vi "test_CRIO daqmx PWM.vi"() -> ()   [LabVIEW 2023]
uses:
  DIO/DO DAQmx PWM CFG/DO DAQmx PWM CFG.lvclass
  Measure and Stimulus Subsystems/Measure and Stimulus Subsystems.lvclass
  DIO/Virtual DIO/Virt PWM Generator/Virt DAQmx PWM Generator.lvclass
panel:
  out "Iteration":i32
  in  "Stop":bool
  out "Error Out":errorcluster
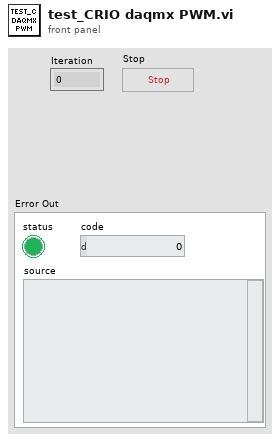
[diagram p1: front panel]
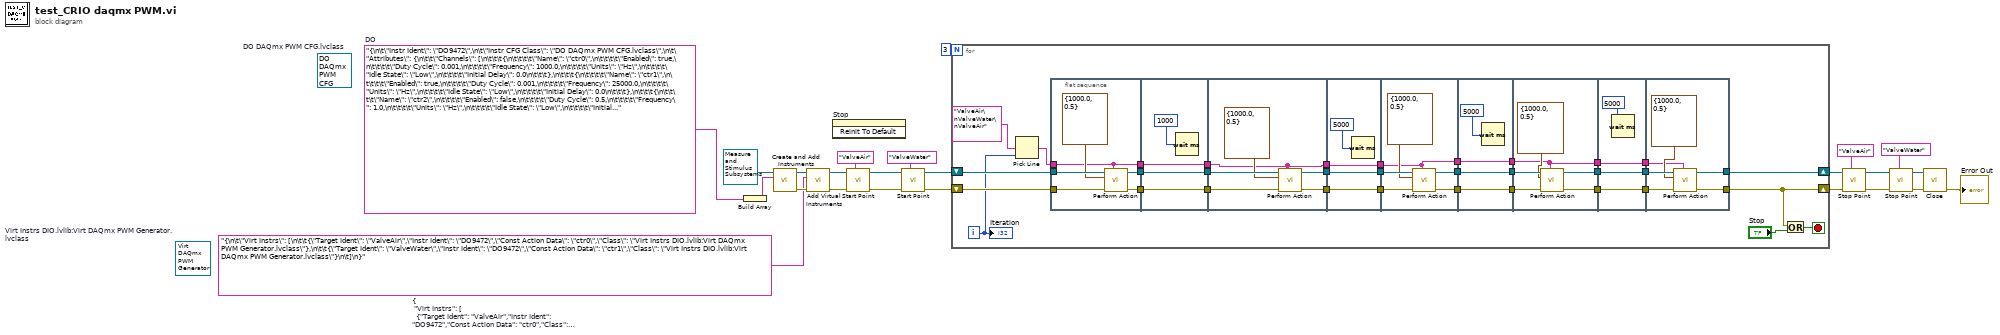
[diagram p0: block diagram]
diagram:
  (unwired) refnum<class "Virt DAQmx PWM Generator.lvclass"> refnum  # Virt Instrs DIO.lvlib:Virt DAQmx PWM Generator.lvclass
  (unwired) refnum<class "DO DAQmx PWM CFG.lvclass"> refnum  # DO DAQmx PWM CFG.lvclass
  w16 = "{\n\t\"Instr Ident\": \"DO9472\",\n\t\"Instr CFG Class\": \"DO DAQmx PWM CFG.lvclass\",\n\t\"Attributes\": {\n\t\t\"Channels\": [\n\t\t\t{\n\t\t\t\t\"Name\": \"ctr0\",\n\t\t\t\t\"Enabled\": true,\n\t\t\t\t\"Duty Cycle\": 0.001,\n\t\t\t\t\"Frequency\": 1000.0,\n\t\t\t\t\"Units\": \"Hz\",\n\t\t\t\t\"Idle State\": \"Low\",\n\t\t\t\t\"Initial Delay\": 0.0\n\t\t\t},\n\t\t\t{\n\t\t\t\t\"Name\": \"ctr1\",\n\t\t\t\t\"Enabled\": true,\n\t\t\t\t\"Duty Cycle\": 0.001,\n\t\t\t\t\"Frequency\": 25000.0,\n\t\t\t\t\"Units\": \"Hz\",\n\t\t\t\t\"Idle State\": \"Low\",\n\t\t\t\t\"Initial Delay\": 0.0\n\t\t\t},\n\t\t\t{\n\t\t\t\t\"Name\": \"ctr2\",\n\t\t\t\t\"Enabled\": false,\n\t\t\t\t\"Duty Cycle\": 0.5,\n\t\t\t\t\"Frequency\": 1.0,\n\t\t\t\t\"Units\": \"Hz\",\n\t\t\t\t\"Idle State\": \"Low\",\n\t\t\t\t\"Initial Delay\": 0.0\n\t\t\t},\n\t\t\t{\n\t\t\t\t\"Name\": \"ctr3\",\n\t\t\t\t\"Enabled\": false,\n\t\t\t\t\"Duty Cycle\": 0.5,\n\t\t\t\t\"Frequency\": 1.0,\n\t\t\t\t\"Units\": \"Hz\",\n\t\t\t\t\"Idle State\": \"Low\",\n\t\t\t\t\"Initial Delay\": 0.0\n\t\t\t}\n\t\t],\n\t\t\"Timing\": {\n\t\t\t\"Samples per Channel\": 1000,\n\t\t\t\"Sample Mode\": \"Continuous Samples\",\n\t\t\t\"Sample Rate\": 0.0,\n\t\t\t\"Sample Clock Source\": \"Implicit\",\n\t\t\t\"Active Edge\": \"Rising\"\n\t\t},\n\t\t\"Trigger\": {\n\t\t\t\"Trigger Type\": \"No Trigger\"\n\t\t}\n\t}\n}"  # DO
  w1 = "{\n\t\"Virt Instrs\": [\n\t\t{\"Target Ident\": \"ValveAir\",\"Instr Ident\": \"DO9472\",\"Const Action Data\": \"ctr0\",\"Class\": \"Virt Instrs DIO.lvlib:Virt DAQmx PWM Generator.lvclass\"},\n\t\t{\"Target Ident\": \"ValveWater\",\"Instr Ident\": \"DO9472\",\"Const Action Data\": \"ctr1\",\"Class\": \"Virt Instrs DIO.lvlib:Virt DAQmx PWM Generator.lvclass\"}\n\t]\n}"  # { 	"Virt Instrs": [ 		{"Target Ident": "ValveAir","Instr Ident": "DO9472","Const Action Data": "ctr0","Class": "Virt Instrs DIO.lvlib:Virt DAQmx PWM Generator.lvclass"}, 		{"Target Ident": "ValveWater","Instr Ident": "DO9472","Const Action Data": "ctr1","Class": "Virt Instrs DIO.lvlib:Virt DAQmx PWM Generator.lvclass"} 	] }
  n1 = Build Array(w16) -> (w2:string[])
  n2 = call "Create and Add Instruments.vi"("Physical Intr CFGs"=w2, "MSS in"=refnum<class "Measure and Stimulus Subsystems.lvclass"> refnum) -> ("Error Out"=w24:errorcluster, "MSS out"=w9:refnum<class "Measure and Stimulus Subsystems.lvclass">)  [unwired: 8 in]
  n3 = call "Add Virtual Instruments.vi"("error in"=w24, "<JSON CFG>"=w1, "MSS in"=w9) -> ("error out"=w11:errorcluster, "MSS out"=w10:refnum<class "Measure and Stimulus Subsystems.lvclass">)  [unwired: 7 in]
  n4 = invoke on="Stop" class="Bool (strict)" method="Reinit To Default"() -> ()  [unwired: 3 in, 3 out]
  n5 = call "Start Point.vi"("Position Ident"="ValveAir" ("Target Identifier"), "error in"=w11, "MSS in"=w10) -> ("error out"=w18:errorcluster, "MSS out"=w14:refnum<class "Measure and Stimulus Subsystems.lvclass">)  [unwired: 7 in]
  n6 = call "Start Point.vi"("Position Ident"="ValveWater" ("Target Ident"), "error in"=w18, "MSS in"=w14) -> ("error out"=w15:errorcluster, "MSS out"=w13:refnum<class "Measure and Stimulus Subsystems.lvclass">)  [unwired: 7 in]
  n7 = for {
    N: 3 -> [_]
    shift-right: [w53] -> w20
    shift-left: w15 -> [w57]
    shift-right: [w52] -> w22
    shift-left: w13 -> [w54]
    i -> [w35]
    stop <- w55 stop-if-true
    n8 = Pick Line(multi-line string="ValveAir\nValveWater\nValveAir" ("Target Identifier"), line index=w35) -> (output string=w33:string)  [unwired: 1 in]
    n9 = flat-sequence {
      tunnel: w54 -> [w61]
      tunnel: w57 -> [w63]
      tunnel: [w62] -> w45
      tunnel: [w60] -> w43
      tunnel: w33 -> [w58]
      tunnel: [w58] -> w31
      tunnel: w45 -> [w67]
      tunnel: [w67] -> w44
      tunnel: w43 -> [w66]
      tunnel: [w66] -> w42
      tunnel: [w64] -> w32
      tunnel: w31 -> [w64]
      tunnel: [w72] -> w41
      tunnel: [w70] -> w39
      tunnel: w44 -> [w73]
      tunnel: w42 -> [w71]
      tunnel: w32 -> [w68]
      tunnel: [w68] -> w29
      tunnel: w41 -> [w77]
      tunnel: [w77] -> w40
      tunnel: w39 -> [w76]
      tunnel: [w76] -> w38
      tunnel: [w74] -> w30
      tunnel: w29 -> [w74]
      tunnel: w40 -> [w83]
      tunnel: w38 -> [w82]
      tunnel: [w81] -> w51
      tunnel: [w80] -> w50
      tunnel: w30 -> [w78]
      tunnel: [w78] -> w27
      tunnel: w51 -> [w87]
      tunnel: w50 -> [w86]
      tunnel: [w87] -> w49
      tunnel: [w86] -> w48
      tunnel: [w84] -> w28
      tunnel: w27 -> [w84]
      tunnel: w49 -> [w93]
      tunnel: w48 -> [w91]
      tunnel: [w92] -> w47
      tunnel: [w90] -> w46
      tunnel: w28 -> [w88]
      tunnel: [w88] -> w25
      tunnel: w47 -> [w97]
      tunnel: w46 -> [w96]
      tunnel: [w97] -> w37
      tunnel: [w96] -> w36
      tunnel: [w94] -> w26
      tunnel: w25 -> [w94]
      tunnel: [w100] -> w52
      tunnel: [w102] -> w53
      tunnel: w37 -> [w103]
      tunnel: w36 -> [w101]
      tunnel: w26 -> [w98]
      frame #0 {
        n10 = call "Perform Action.vi"("Point Ident"=w58, "error in"=w63, "Input"=cluster{"Frequency":dbl, "Duty Cycle":dbl} {"Frequency"=1000.0, "Duty Cycle"=0.5} ("PWM Pams"), "MSS in"=w61) -> ("error out"=w62:errorcluster, "MSS out"=w60:refnum<class "Measure and Stimulus Subsystems.lvclass">)  [unwired: 5 in, 1 out]
      }
      frame #1 {
        n11 = Wait (ms)(milliseconds to wait=u32 1000) -> ()  [unwired: 1 out]
      }
      frame #2 {
        n12 = call "Perform Action.vi"("Point Ident"=w68, "error in"=w73, "Input"=cluster{"Frequency":dbl, "Duty Cycle":dbl} {"Frequency"=1000.0, "Duty Cycle"=0.5} ("PWM Pams"), "MSS in"=w71) -> ("error out"=w72:errorcluster, "MSS out"=w70:refnum<class "Measure and Stimulus Subsystems.lvclass">)  [unwired: 5 in, 1 out]
      }
      frame #3 {
        n13 = Wait (ms)(milliseconds to wait=u32 5000) -> ()  [unwired: 1 out]
      }
      frame #4 {
        n14 = call "Perform Action.vi"("Point Ident"=w78, "error in"=w83, "Input"=cluster{"Frequency":dbl, "Duty Cycle":dbl} {"Frequency"=1000.0, "Duty Cycle"=0.5} ("PWM Pams"), "MSS in"=w82) -> ("error out"=w81:errorcluster, "MSS out"=w80:refnum<class "Measure and Stimulus Subsystems.lvclass">)  [unwired: 5 in, 1 out]
      }
      frame #5 {
        n15 = Wait (ms)(milliseconds to wait=u32 5000) -> ()  [unwired: 1 out]
      }
      frame #6 {
        n16 = call "Perform Action.vi"("Point Ident"=w88, "error in"=w93, "Input"=cluster{"Frequency":dbl, "Duty Cycle":dbl} {"Frequency"=1000.0, "Duty Cycle"=0.5} ("PWM Pams"), "MSS in"=w91) -> ("error out"=w92:errorcluster, "MSS out"=w90:refnum<class "Measure and Stimulus Subsystems.lvclass">)  [unwired: 5 in, 1 out]
      }
      frame #7 {
        n17 = Wait (ms)(milliseconds to wait=u32 5000) -> ()  [unwired: 1 out]
      }
      frame #8 {
        n18 = call "Perform Action.vi"("Point Ident"=w98, "error in"=w103, "Input"=cluster{"Frequency":dbl, "Duty Cycle":dbl} {"Frequency"=1000.0, "Duty Cycle"=0.5} ("PWM Pams"), "MSS in"=w101) -> ("error out"=w102:errorcluster, "MSS out"=w100:refnum<class "Measure and Stimulus Subsystems.lvclass">)  [unwired: 5 in, 1 out]
      }
    }
    n19 = Or(x=w53, y="Stop") -> (x .or. y?=w55:bool)
    "Iteration" <- w35
  }
  n20 = call "Stop Point.vi"("Point Ident"="ValveAir" ("Target Identifier"), "error in"=w20, "MSS in"=w22) -> ("error out"=w23:errorcluster, "MSS out"=w7:refnum<class "Measure and Stimulus Subsystems.lvclass">)  [unwired: 7 in]
  n21 = call "Stop Point.vi"("Point Ident"="ValveWater" ("Target Ident"), "error in"=w23, "MSS in"=w7) -> ("error out"=w8:errorcluster, "MSS out"=w6:refnum<class "Measure and Stimulus Subsystems.lvclass">)  [unwired: 7 in]
  n22 = call "Close.vi"("error in"=w8, "MSS in"=w6) -> ("error out"=→"Error Out":errorcluster)  [unwired: 8 in, 1 out]
